vi "io.command-parser.DI.vi"(8 "error in (no error)":errorcluster, 10 "Reponse in":string="{ß\u0005\u0001\u0016\u0010\u0001\u0004\u0002ß}", 11 "IoConf out":T1={"ADDR"=0, "Label"="", "Type"=enum."DI", "Mode"=enum."RIO", "Value"="", "Tags"="", "calibration"=[]} {"calibration"."Y" format="%#.3f"; "calibration"."X" format="%#.3f"; "ADDR" format="%04d"}) -> (0 "error out":errorcluster, 1 "dports":bool[](array[boolean]), 2 "DI out":dbl)   [LabVIEW 2024]
uses:
  controls/IONode.ctl
  controls/type.address.ctl
  controls/enum.io.type.ctl
  controls/enum.io.mode.ctl
  controls/typeXyPoint.ctl
panel:
  out "size(s)":i32
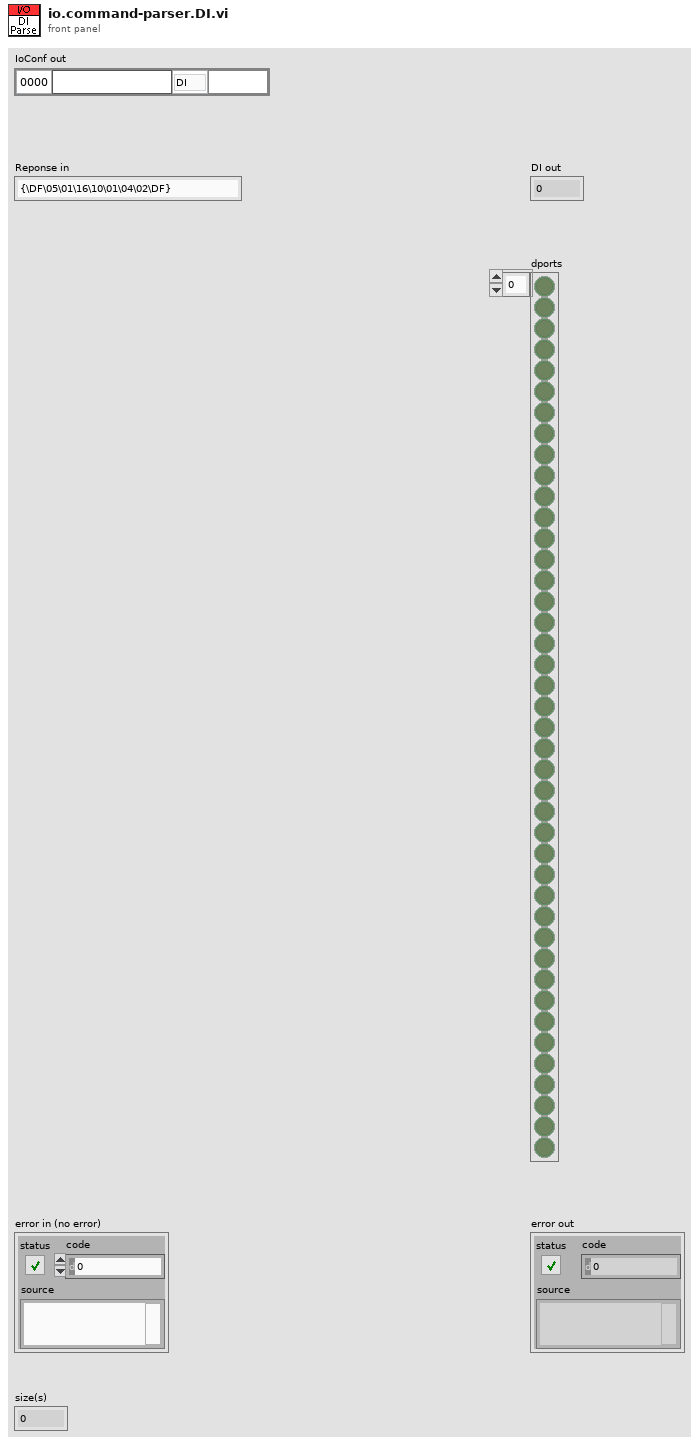
[diagram p1: front panel]
types:
  T1 = typedef "IONode.ctl" = cluster{"ADDR":T2, "Label":string, "Type":T3, "Mode":T4, "Value":string, "Tags":string, "calibration":T5[]}
  T2 = typedef "type.address.ctl" = u16
  T3 = typedef "enum.io.type.ctl" = enum16{"Type", "DI", "DO", "AI", "AO", "VL", "BUF"}
  T4 = typedef "enum.io.mode.ctl" = enum16{"Mode", "RIO", "SIM"}
  T5 = typedef "typeXyPoint.ctl" = cluster{"X":dbl, "Y":dbl}
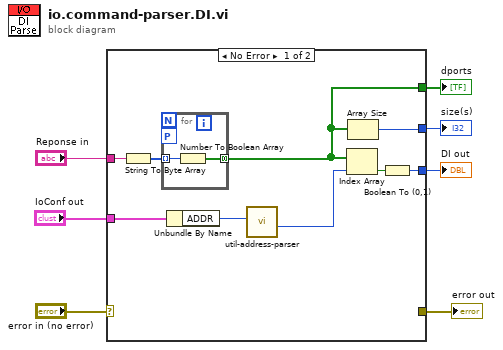
[diagram p0: block diagram]
diagram:
  n1 = case shown="No Error" "error in (no error)" {
    selector: "error in (no error)" -> [_ w19]
    tunnel: "Reponse in" -> [w16 _]
    tunnel: "IoConf out" -> [w9 _]
    tunnel: [w13 _] -> w6
    tunnel: [w12 _] -> w5
    tunnel: [w11 _] -> w4
    tunnel: [_ w19] -> w2
    frame No Error {
      n2 = String To Byte Array(string=w16) -> (unsigned byte array=w14:u8[])
      n3 = for {
        tunnel: w14 -> [w18] mode=indexing
        tunnel: [w17] -> w13 mode=concatenating
        workers-P: _ -> [_]
        n4 = Number To Boolean Array(number=w18) -> (Boolean array=w17:bool[])
      }
      n5 = Unbundle By Name(w9) -> ("ADDR"=w10:T2)
      n6 = call "util-address-parser.vi"("ADDR 2"=w10) -> ("Channel"=w8:u8)  [unwired: 9 in, 1 out]
      n7 = Index Array(array=w13, index=w8) -> (element=w15:bool)
      n8 = Array Size(array=w13) -> (size(s)=w12:i32)
      n9 = Boolean To (0,1)(Boolean=w15) -> (0, 1=w11:i16)
    }
    frame Error {
    }
  }
  "error out" <- w2
  "DI out" <- w4
  "dports" <- w6
  "size(s)" <- w5
